vi "Select Routing Objects.vi"(10 "Controller":refnum<class "Controller.lvclass">, 11 "Inputs":refnum<class "Processing.lvclass">) -> (3 "Updated Inputs":refnum<class "Processing.lvclass">, 5 "Controller?":bool, 7 "Trace Message":string)   [LabVIEW 2020, in "HTTP Server.lvlib" / "Server.lvclass"]
uses:
  Server.lvclass
  Server.lvclass/Server.ctl
  Controller/Controller.lvclass
  C:/dev/lv20CE/relink/lv-http-server/HTTP Server/Controller/Controller.lvclass
  C:/dev/lv20CE/relink/lv-http-server/HTTP Server/Handler/Handler.lvclass
  Processing/Processing.lvclass
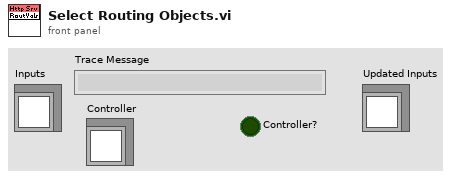
[diagram p1: front panel]
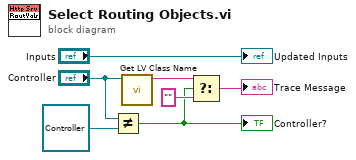
[diagram p0: block diagram]
diagram:
  n1 = Not Equal?(x="Controller", y=refnum<class "Controller.lvclass"> refnum) -> (x != y?=w4:bool)
  "Controller?" <- w4
  n2 = call <vilib>:"Get LV Class Name.vi"("object"="Controller") -> ("class name"=w6:string)  [unwired: 9 in, 1 out]
  n3 = Select(t=w6, s=w4, f="") -> (s? t:f=→"Trace Message":string)
  "Updated Inputs" <- "Inputs"
